vi "CC Rd Wr Script.vi"(8 "error in (no error)":errorcluster, 9 "Script Path":path, 10 "Action":T1, 11 "Script":T2) -> (0 "error out":errorcluster, 1 "Syntax Errors":string, 2 "Script List":string[](array[string]), 3 "Script":T2, 4 "Script Ok?":bool, 5 "Script Path":path)   [LabVIEW 2021]
uses:
  typedefs/CC cluster Script.ctl
  typedefs/CC Script Step.ctl
  typedefs/CC enum Script Action.ctl
  CC Rd Wr Script Action.ctl
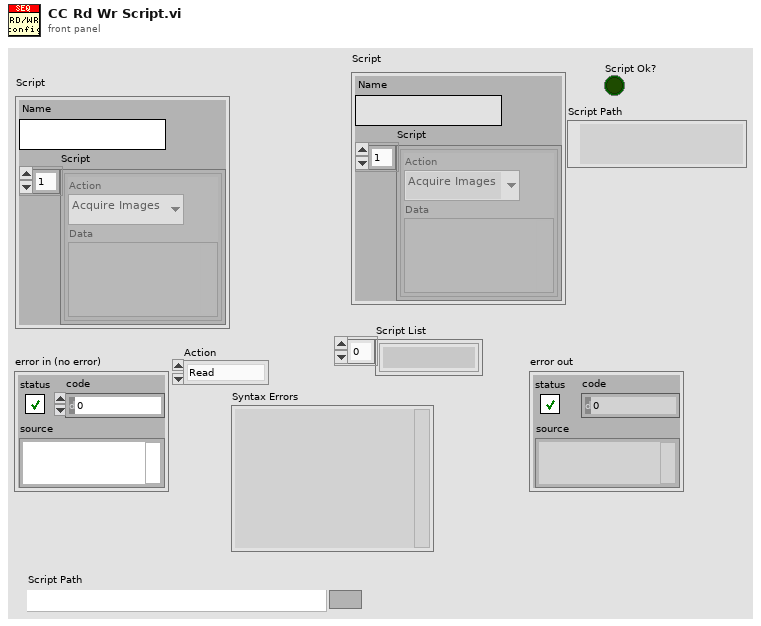
[diagram p1: front panel]
types:
  T1 = typedef "CC Rd Wr Script Action.ctl" = enum16{"Read", "Write", "List", "Delete"}
  T2 = typedef "CC cluster Script.ctl" = cluster{"Name":string, "Script":T3[]}
  T3 = typedef "CC Script Step.ctl" = cluster{"Action":T4, "Data":variant}
  T4 = typedef "CC enum Script Action.ctl" = enum16{"Noop", "Define Object", "Define Exposure", "Define Dithering", "Acquire Images", "Set Filter Wheel", "Telescope Home", "Telescope Move", "Telescope RA DEC", "Focus Move Relative", "Focus Move Absolute", "Focus Set Home", "Macro", "Pause", "Ask User", "Define Random Dither"}
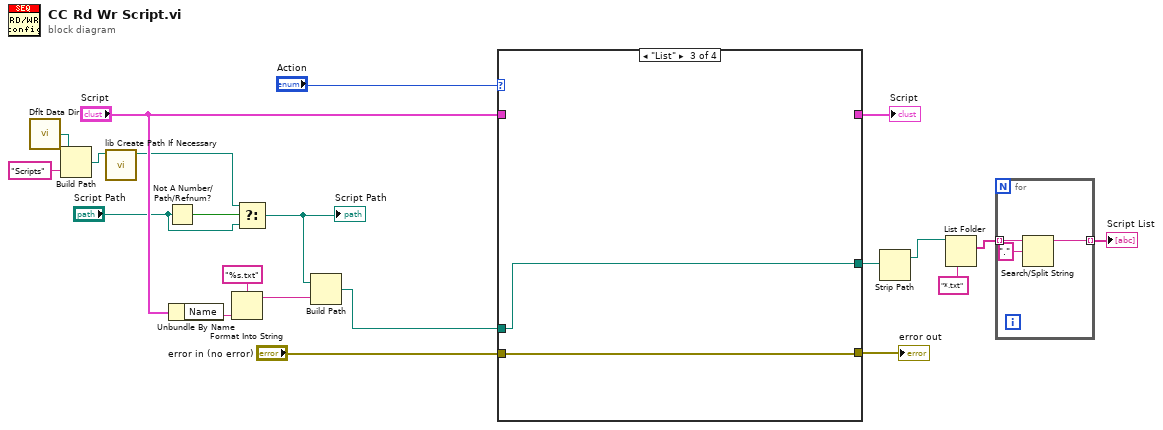
[diagram p0: block diagram]
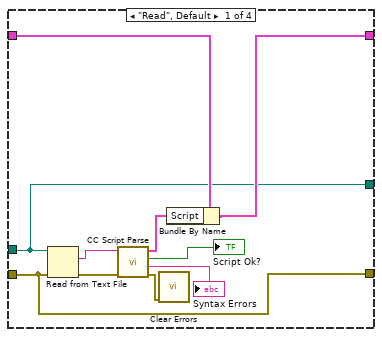
[diagram p2: hidden frame]
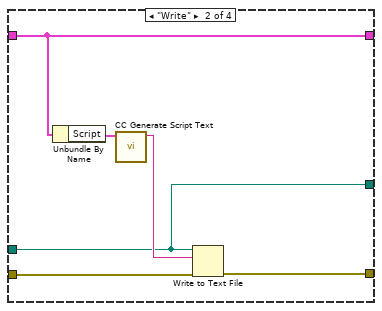
[diagram p3: hidden frame]
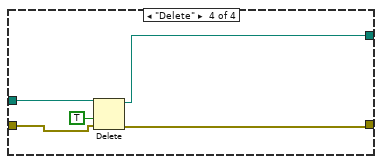
[diagram p4: hidden frame]
diagram:
  n1 = call <vilib>:"Dflt Data Dir.vi"() -> ("App:Default Data Directory"=w12:path)
  n2 = Build Path(base path=w12, name or relative path="Scripts") -> (appended path=w10:path)
  n3 = call "lib Create Path If Necessary.vi"("path"=w10) -> ("path out"=w3:path)  [unwired: 10 in]
  n4 = Not A Number/Path/Refnum?(number/path/refnum="Script Path") -> (NaN/Path/Refnum?=w4:bool)
  n5 = Unbundle By Name("Script") -> ("Name"=w15:string)
  n6 = Format Into String(format string="%s.txt" ("name or relative path"), w15) -> (resulting string=w13:string)  [unwired: 2 in, 1 out]
  n7 = Select(t=w3, s=w4, f="Script Path") -> (s? t:f=w2:path)
  "Script Path" <- w2
  n8 = Build Path(base path=w2, name or relative path=w13) -> (appended path=w19:path)
  n9 = case shown="\"List\"" "Action" {
    tunnel: "error in (no error)" -> [w31 w37 w38 w42]
    tunnel: "Script" -> [w28 w35 _ _]
    tunnel: w19 -> [w25 w32 w39 w44]
    tunnel: [w31 w36 w38 w41] -> w18
    tunnel: [w26 w35 _ _] -> w17
    tunnel: [w25 w32 w39 w40] -> w8
    frame "Read", Default {
      n10 = Read from Text File(file (use dialog)=w25, error in=w31) -> (text=w30:string, error out=w29:errorcluster)  [unwired: 2 in, 2 out]
      n11 = call "CC Script Parse.vi"("error in (no error)"=w29, "Script text"=w30) -> ("error out"=w22:errorcluster, "Syntax Errors"=→"Syntax Errors":string, "Script Ok?"=→"Script Ok?":bool, "Script steps"=w27:T3[])  [unwired: 6 in]
      n12 = call <vilib>:"Clear Errors.vi"("error in (no error)"=w22) -> ()  [unwired: 5 in, 2 out]
      n13 = Bundle By Name(cluster=w28, "Script"=w27) -> (w26:T2)
    }
    frame "Write" {
      n14 = Unbundle By Name(w35) -> ("Script"=w34:T3[])
      n15 = call "CC Generate Script Text.vi"("Script"=w34) -> ("Script String"=w33:string)  [unwired: 9 in, 1 out]
      n16 = Write to Text File(file (use dialog)=w32, text=w33, error in=w37) -> (error out=w36:errorcluster)  [unwired: 1 in, 2 out]
    }
    frame "List" {
    }
    frame "Delete" {
      n17 = Delete(path (use dialog)=w44, confirm (F)=TRUE, error in=w42) -> (deleted path=w40:path, error out=w41:errorcluster)  [unwired: 2 in, 1 out]
    }
  }
  "error out" <- w18
  "Script" <- w17
  n18 = Strip Path(path=w8) -> (stripped path=w7:path)  [unwired: 1 out]
  n19 = List Folder(path=w7, pattern="*.txt") -> (filenames=w6:string[])  [unwired: 2 in, 3 out]
  n20 = for {
    tunnel: w6 -> [w47] mode=indexing
    tunnel: [w45] -> w5 mode=indexing
    n21 = Search/Split String(string=w47, search string/char (-)=".") -> (substring before match=w45:string)  [unwired: 1 in, 2 out]
  }
  "Script List" <- w5
